vi "Force Copy.vi"(8 "error in (no error)":errorcluster, 10 "target":path, 11 "source":path) -> (0 "error out":errorcluster)   [LabVIEW 2016]
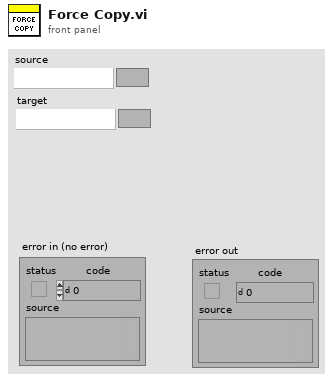
[diagram p1: front panel]
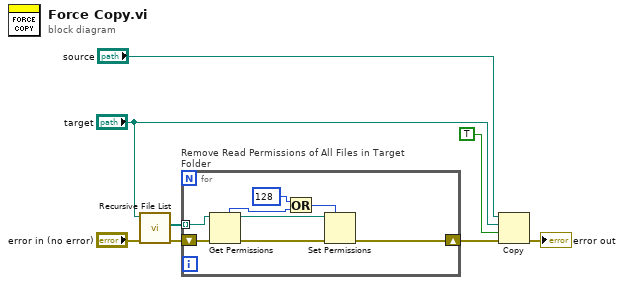
[diagram p0: block diagram]
diagram:
  n1 = call <vilib>:"Recursive File List.vi"("error in (no error)"="error in (no error)", "Folder Path"="target") -> ("error out"=w2:errorcluster, "All Files in Dir"=w1:path[])  [unwired: 5 in, 3 out]
  n2 = for "Remove Read Permissions of All Files in Target Folder" {
    shift-right: [w11] -> w5
    shift-left: w2 -> [w10]
    tunnel: w1 -> [w9] mode=indexing
    n3 = Get Permissions(8:w10, 11:w9) -> (0:w13:errorcluster, 3:w12:path, 5:w15:i16)  [unwired: 2 out]
    n4 = Or(x=i16 128 ("new permissions"), y=w15) -> (x .or. y?=w14:i16)
    n5 = Set Permissions(7:w14, 8:w13, 11:w12) -> (0:w11:errorcluster)  [unwired: 2 in, 1 out]
  }
  n6 = Copy(8:w5, 9:TRUE ("overwrite (F)"), 10:"target", 11:"source") -> (0:→"error out":errorcluster)  [unwired: 1 in, 2 out]
